vi "Init libssh2_knownhost.vi"(8 "error in (no error)":errorcluster) -> (0 "error out":errorcluster, 3 "libssh2_knownhost*":u64 format="%.0x")   [LabVIEW 2013, in "libssh2.lvlib"]
uses:
  libssh2.lvlib
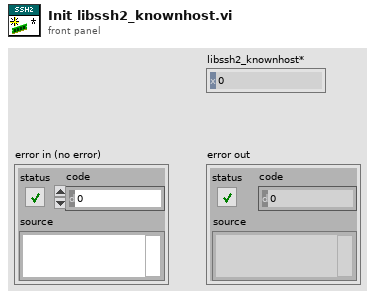
[diagram p1: front panel]
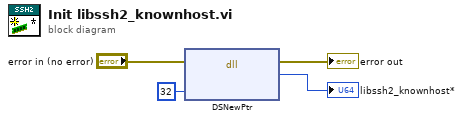
[diagram p0: block diagram]
diagram:
  n1 = dll-call lib="LabVIEW" fn="DSNewPtr"(error in="error in (no error)", "size"=i64 32) -> (error out=→"error out":errorcluster, "return type"=→"libssh2_knownhost*":u64)  [unwired: 3 in, 1 out]
